vi "ma-resample unevenly sampled input (coerce).vi"(0 "X-array in":dbl[](array[numeric]) format="%.2p", 5 "Y-array in":dbl[](array[numeric]) format="%.2p", 7 "dt":dbl=1.0 format="%.2p", 9 "t0":dbl format="%.2p", 11 "error in":errorcluster) -> (4 "X-array out":dbl[](array[numeric]) format="%.2p", 6 "Y-array out":dbl[](array[numeric]) format="%.2p", 8 "evenly sampled waveform out":waveform(dbl), 10 "used t0":dbl format="%.2p", 14 "t0 adjusted warning":bool, 15 "error out":errorcluster)   [LabVIEW 2020, in "NI_MAPro.lvlib"]
doc: "This VI re-samples an unevenly sampled input signal to an evenly sampled waveform according to specified t0 and dt. If the specified t0 value is less than the first value of input X-array (that is the timestamp of the first input sample), then the VI will coerce t0 to the first valid value (greater than X(0)) that also fulfill the relation:\n\nT0_adjusted - t0_in = n * dt_in\n\nThis guarranty that any later comparison of waveforms will be correct with repsect to absolute time."
uses:
  NI_MAPro.lvlib
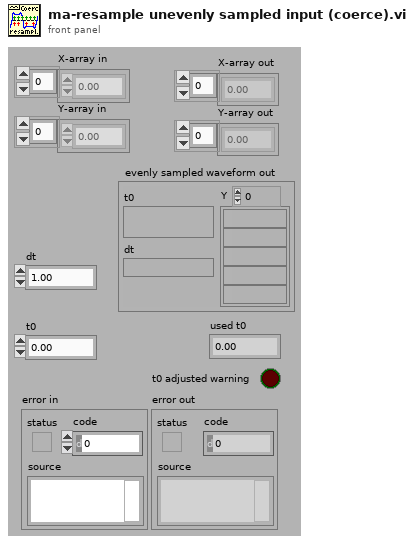
[diagram p1: front panel]
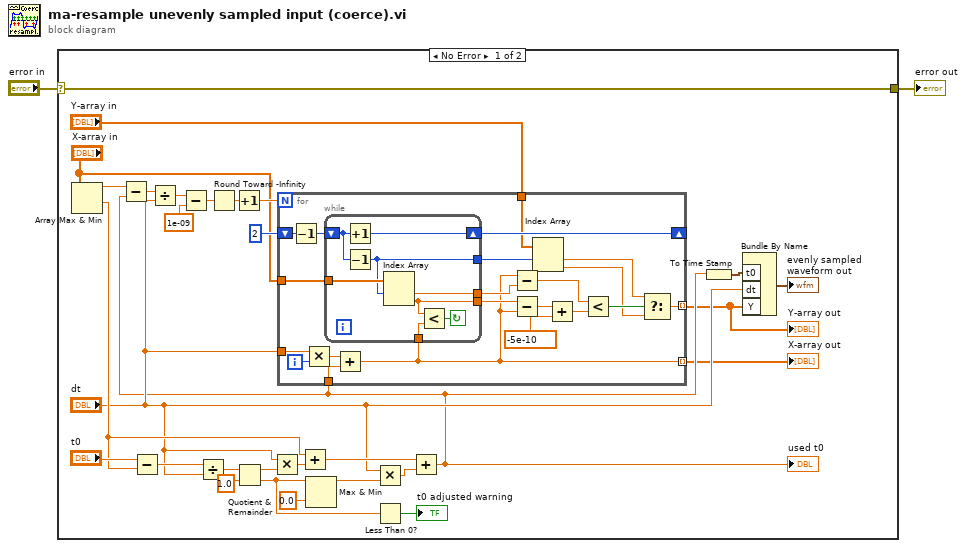
[diagram p0: block diagram]
diagram:
  n1 = case shown="No Error" "error in" {
    selector: "error in" -> [w4 w62]
    tunnel: [w4 w62] -> w1
    frame No Error {
      n2 = Array Max & Min(array="X-array in") -> (max value=w17:dbl, min value=w14:dbl)  [unwired: 2 out]
      n3 = Subtract(x="t0", y=w14) -> (x-y=w29:dbl)
      n4 = Divide(x=w29, y="dt") -> (x/y=w31:dbl)
      n5 = Quotient & Remainder(x=w31, y=1.0) -> (x-y*floor(x/y)=w20:dbl, floor(x/y)=w22:dbl)
      n6 = Multiply(x="dt", y=w20) -> (x*y=w28:dbl)
      n7 = Add(x=w14, y=w28) -> (x+y=w25:dbl)
      n8 = Max & Min(x=w22, y=0.0) -> (max(x,y)=w24:dbl)  [unwired: 1 out]
      n9 = Multiply(x="dt", y=w24) -> (x*y=w27:dbl)
      n10 = Less Than 0?(x=w22) -> (x < 0?=→"t0 adjusted warning":bool)
      n11 = Add(x=w25, y=w27) -> (x+y=w12:dbl)
      "used t0" <- w12
      n12 = Subtract(x=w17, y=w12) -> (x-y=w18:dbl)
      n13 = Divide(x=w18, y="dt") -> (x/y=w11:dbl)
      n14 = Subtract(x=w11, y=1e-09) -> (x-y=w9:dbl)
      n15 = Round Toward -Infinity(1:w9) -> (0:w16:dbl)
      n16 = Increment(x=w16) -> (x+1=w15:dbl)
      n17 = for {
        N: w15 -> [_]
        tunnel: "dt" -> [w52]
        tunnel: w12 -> [w50]
        tunnel: "X-array in" -> [w49]
        shift-right: [w47] -> _
        shift-left: 2 -> [w48]
        tunnel: [w40] -> w5 mode=indexing
        tunnel: "Y-array in" -> [w45]
        tunnel: [w36] -> w6 mode=indexing
        i -> [w53]
        n18 = Decrement(x=w48) -> (x-1=w46:i32)
        n19 = Multiply(x=w52, y=w53) -> (x*y=w51:dbl)
        n20 = Add(x=w51, y=w50) -> (x+y=w40:dbl)
        n21 = while {
          tunnel: w49 -> [w61]
          shift-right: [w59] -> w47
          shift-left: w46 -> [w56]
          tunnel: w40 -> [w60]
          tunnel: [w55] -> w44
          tunnel: [w57] -> w41
          tunnel: [w58] -> w42
          stop <- w54 continue-if-true
          n22 = Increment(x=w56) -> (x+1=w59:i32)
          n23 = Decrement(x=w56) -> (x-1=w55:i32)
          n24 = Index Array(array=w61, index #1=w55) -> (element #1=w57:dbl, element #2=w58:dbl)  [unwired: 1 in]
          n25 = Less?(x=w58, y=w60) -> (x < y?=w54:bool)
        }
        n26 = Subtract(x=w40, y=w41) -> (x-y=w43:dbl)
        n27 = Subtract(x=w42, y=w40) -> (x-y=w34:dbl)
        n28 = Index Array(array=w45, index #1=w44) -> (element #1=w38:dbl, element #2=w37:dbl)  [unwired: 1 in]
        n29 = Add(x=w34, y=-5e-10) -> (x+y=w35:dbl)
        n30 = Less?(x=w43, y=w35) -> (x < y?=w39:bool)
        n31 = Select(t=w38, s=w39, f=w37) -> (s? t:f=w36:dbl)
      }
      "X-array out" <- w5
      "Y-array out" <- w6
      n32 = To Time Stamp(1:w12) -> (0:w3:timestamp)
      n33 = Bundle By Name("t0"=w3, "dt"="dt", "Y"=w6) -> (→"evenly sampled waveform out":waveform(dbl))  [unwired: 1 in]
    }
    frame Error {
    }
  }
  "error out" <- w1
